vi "Ctor.vi"(8 "error in (no error)":errorcluster) -> (0 "error out":errorcluster, 3 "Unit Of Work out":refnum<class "Unit Of Work Session.lvclass">)   [LabVIEW 2020, in "Conditum.lvlib" / "Unit Of Work Session.lvclass"]
uses:
  Unit Of Work Session.lvclass
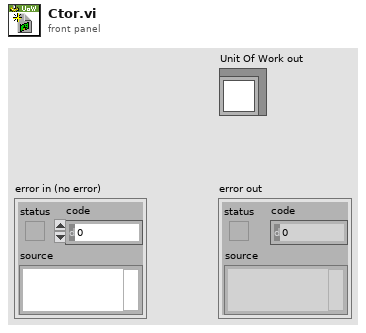
[diagram p1: front panel]
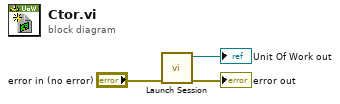
[diagram p0: block diagram]
diagram:
  n1 = call "Launch Session.vi"("error in (no error)"="error in (no error)") -> ("error out"=→"error out":errorcluster, "Unit Of Work out"=→"Unit Of Work out":refnum<class "Unit Of Work Session.lvclass">)  [unwired: 9 in]
